vi "svx_Parse Format String.vi"(11 "Format string":string) -> (0 "trailing zeros":bool, 1 "Precision Type":u16(ring) items=["Digits of precision", "Significant digits"], 2 "Digits":u8=1, 3 "Type":i32(listbox), 4 "Custom Format?":bool)   [LabVIEW 2017, in "SVX Waterfall Graph.xctl"]
uses:
  <vilib>/addons/_XControls/Waterfall Graph/SVX Waterfall Graph.xctl
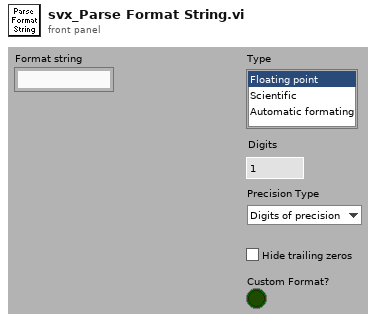
[diagram p1: front panel]
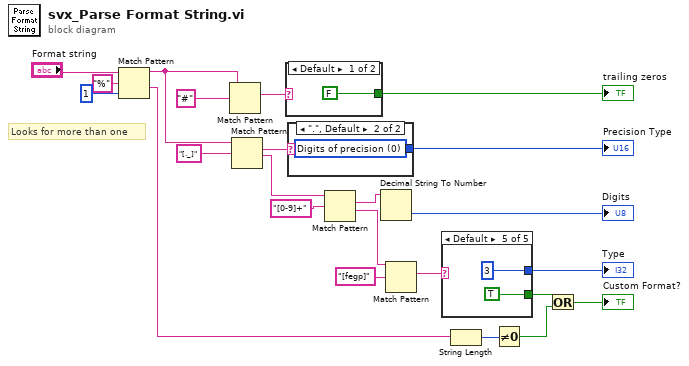
[diagram p0: block diagram]
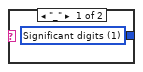
[diagram p2: hidden frame]
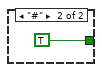
[diagram p3: hidden frame]
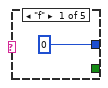
[diagram p4: hidden frame]
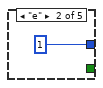
[diagram p5: hidden frame]
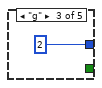
[diagram p6: hidden frame]
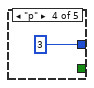
[diagram p7: hidden frame]
diagram:
  # "Looks for more than one"
  n1 = Match Pattern(string="Format string", regular expression="%", offset (0)=1) -> (before substring=w6:string, after substring=w4:string)  [unwired: 2 out]
  n2 = Match Pattern(string=w6, regular expression="#") -> (match substring=w17:string)  [unwired: 1 in, 3 out]
  n3 = Match Pattern(string=w6, regular expression="[._]") -> (match substring=w14:string, after substring=w5:string)  [unwired: 1 in, 2 out]
  n4 = case shown="Default" w17 {
    tunnel: [FALSE ("trailing zeros") TRUE ("trailing zeros")] -> w16
    frame Default {
    }
    frame "#" {
    }
  }
  "trailing zeros" <- w16
  n5 = case shown="\".\", Default" w14 {
    tunnel: [w26 w27] -> w13
    frame "_" {
      w26 = u16 1 items=["Digits of precision", "Significant digits"] ("Precision Type")
    }
    frame ".", Default {
      w27 = u16 0 items=["Digits of precision", "Significant digits"] ("Precision Type")
    }
  }
  "Precision Type" <- w13
  n6 = Match Pattern(string=w5, regular expression="[0-9]+") -> (match substring=w10:string, after substring=w9:string)  [unwired: 1 in, 2 out]
  n7 = Decimal String To Number(string=w10) -> (number=→"Digits":i32)  [unwired: 2 in, 1 out]
  n8 = Match Pattern(string=w9, regular expression="[fegp]" ("search string")) -> (match substring=w22:string)  [unwired: 1 in, 3 out]
  n9 = case shown="Default" w22 {
    tunnel: [0 ("Type") 1 ("Type") 2 ("Type") 3 ("Type") 3 ("Type")] -> w21
    tunnel: [_ _ _ _ TRUE ("x != 0?")] -> w3
    frame "f" {
    }
    frame "e" {
    }
    frame "g" {
    }
    frame "p" {
    }
    frame Default {
    }
  }
  "Type" <- w21
  n10 = String Length(string=w4) -> (length=w8:i32)
  n11 = Not Equal To 0?(x=w8) -> (x != 0?=w2:bool)
  n12 = Or(x=w3, y=w2) -> (x .or. y?=→"Custom Format?":bool)
